vi "Muninn.vi"() -> ()   [LabVIEW 2025]
uses:
  <vilib>/OPCUA/NI OPC UA Client.lvlib
  <vilib>/Utility/config.llb/NI_LVConfig.lvlib
  <vilib>/Utility/config.llb/Read Key (String).vi
  <vilib>/OPCUA/client/Multiple Read Double.vi
panel:
  in  "Preferences Button":bool
  in  "Remove Button":bool
  in  "Add Button":bool
  in  "Sensors":i32(listbox)
  in  "Stop button":bool
  in  "Start Button":bool
  in  "LoggingIntervall":dbl=1000.0 caption="Logging intervall (ms)"
  out "running":bool
  in  "quit":bool
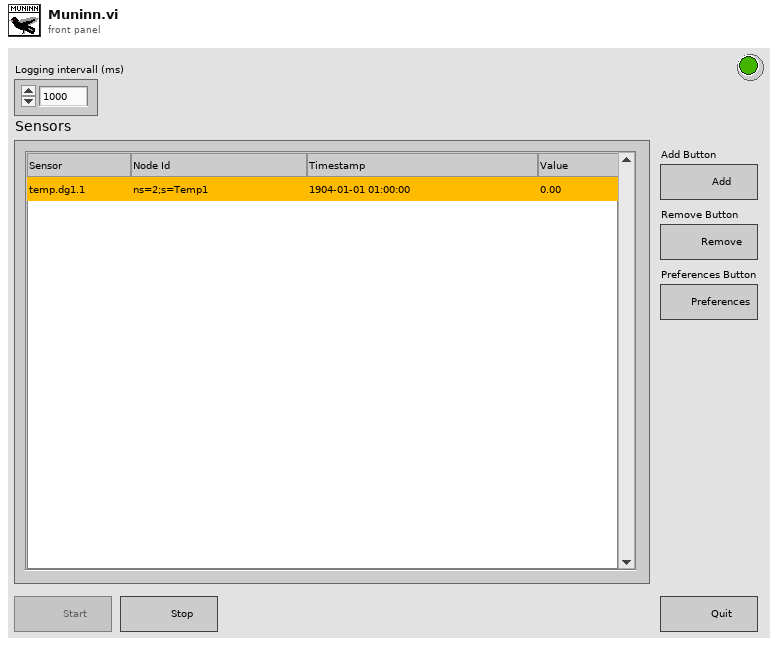
[diagram p1: front panel]
types:
  T1 = enum8{"Enabled", "Disabled", "Disabled and Grayed Out"}
  T2 = typedef "NI_LVConfig.lvlib/Config Data RefNum.ctl" = refnum<k1>
  T3 = typedef "OPC UA Client Refnum.ctl" = refnum<k21>
  T4 = typedef "NodeId.ctl" = string
  T5 = typedef "OPC UA StatusCode.ctl" = u32
  T6 = cluster{"node ID":T4, "value ":dbl, "timestamp":timestamp, "status":T5}[]
  T7 = cluster{"node ID":T4, "value ":dbl, "timestamp":timestamp, "status":T5}
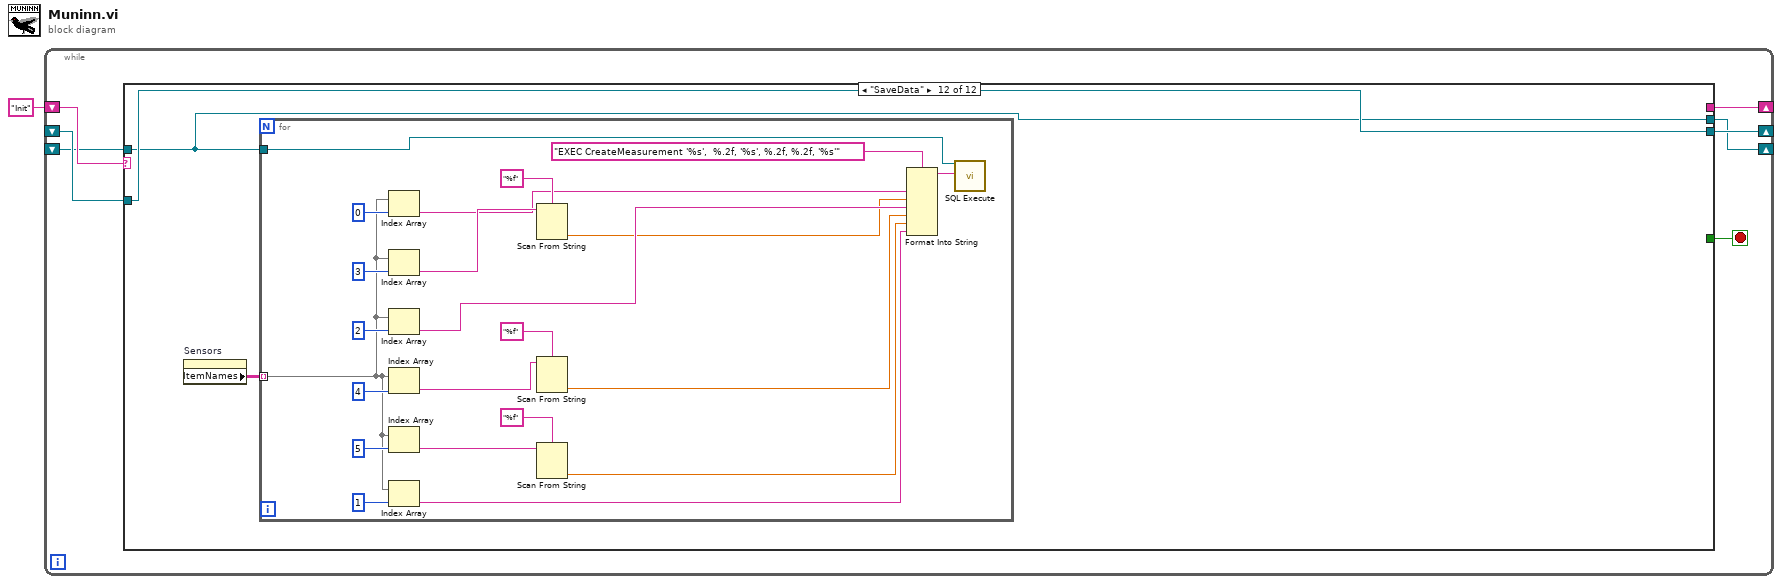
[diagram p0: block diagram]
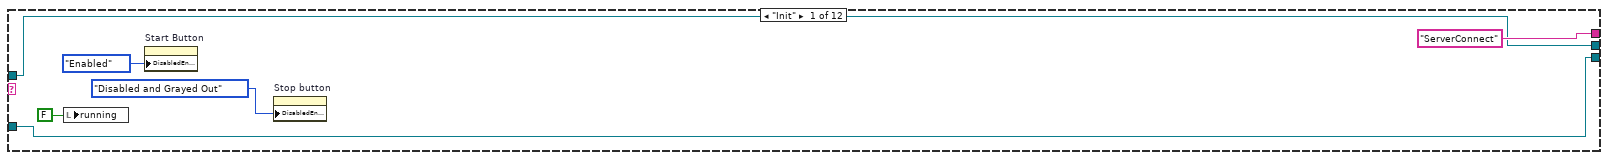
[diagram p2: hidden frame]
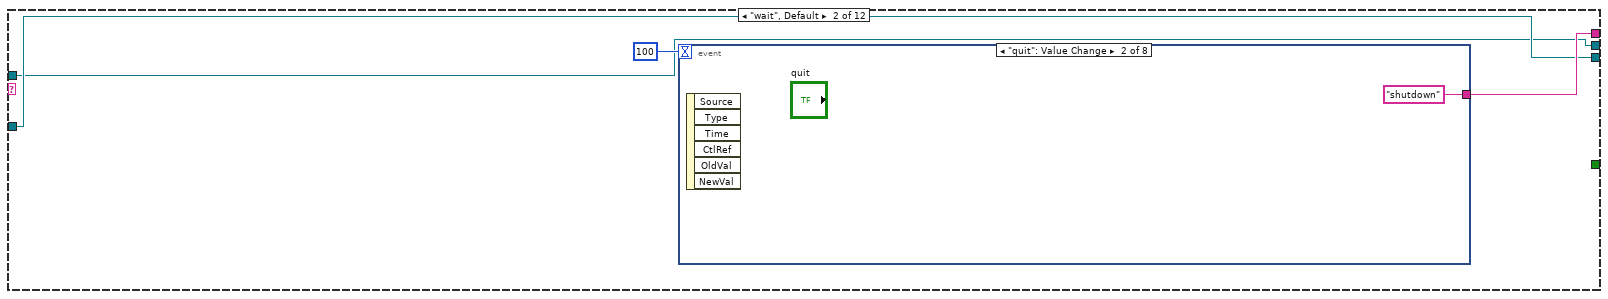
[diagram p3: hidden frame]
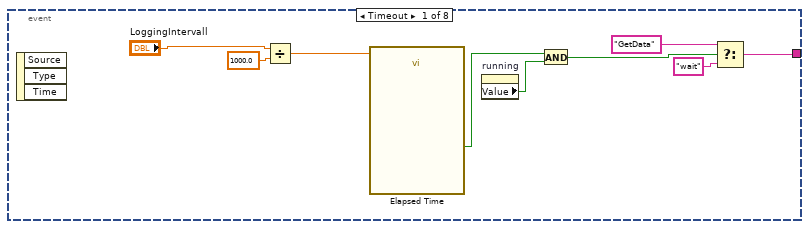
[diagram p4: hidden frame]
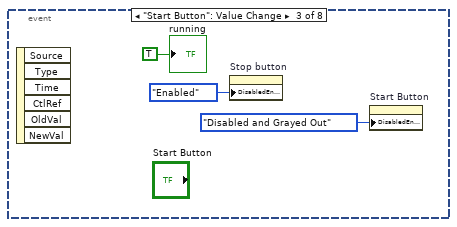
[diagram p5: hidden frame]
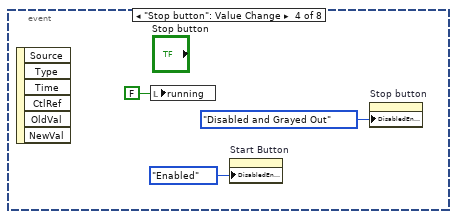
[diagram p6: hidden frame]
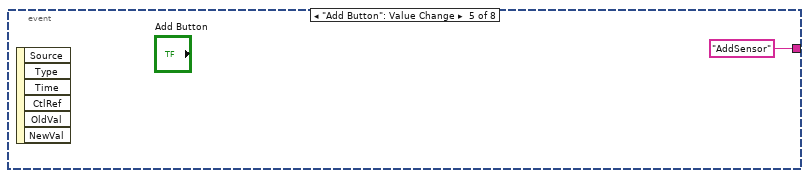
[diagram p7: hidden frame]
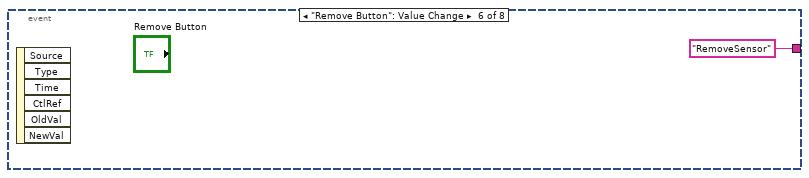
[diagram p8: hidden frame]
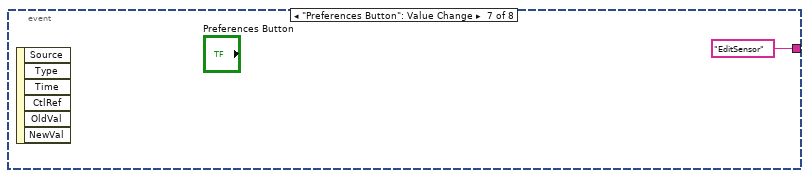
[diagram p9: hidden frame]
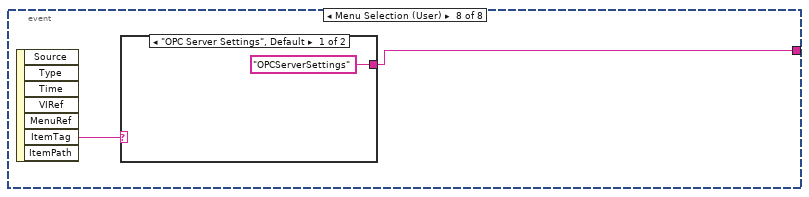
[diagram p10: hidden frame]
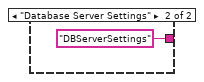
[diagram p11: hidden frame]
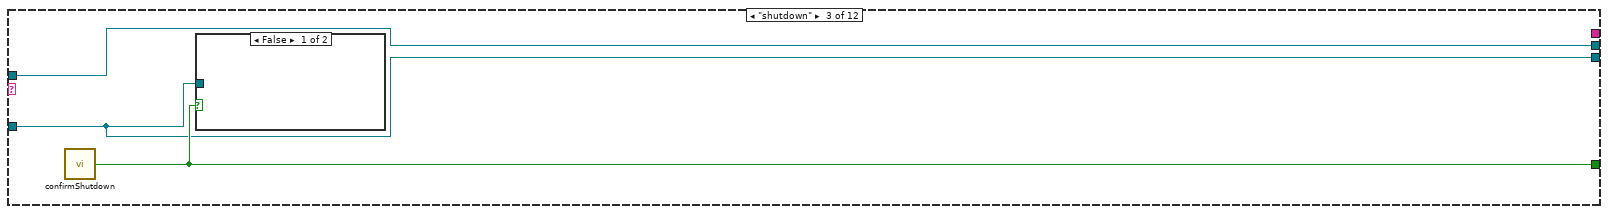
[diagram p12: hidden frame]
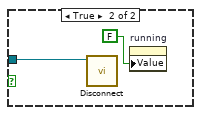
[diagram p13: hidden frame]
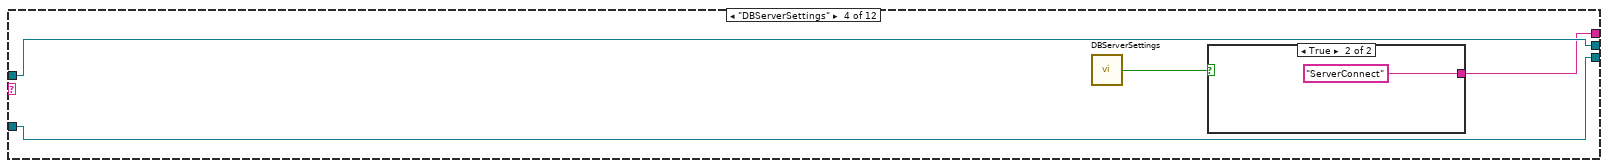
[diagram p14: hidden frame]
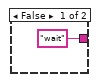
[diagram p15: hidden frame]
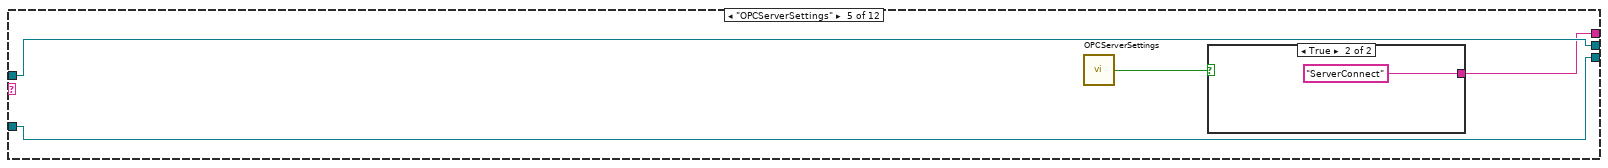
[diagram p16: hidden frame]
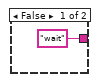
[diagram p17: hidden frame]
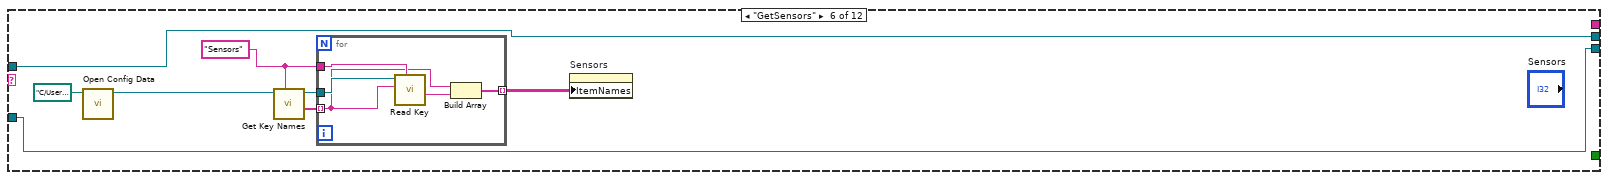
[diagram p18: hidden frame]
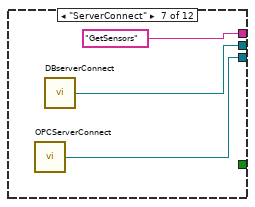
[diagram p19: hidden frame]
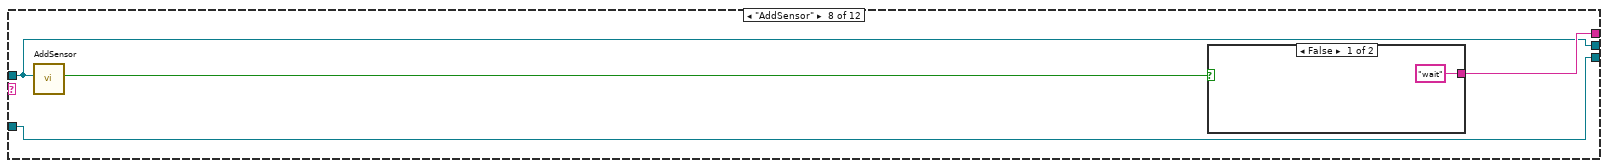
[diagram p20: hidden frame]
diagram:
  n1 = while {
    shift-right: [w7] -> _
    shift-left: "Init" -> [w8]
    shift-right: [w5] -> _
    shift-left: _ -> [w4]
    shift-right: [w3] -> _
    shift-left: _ -> [w2]
    stop <- w6 stop-if-true
    n2 = case shown="\"SaveData\"" w8 {
      tunnel: ["ServerConnect" w17 _ w48 w53 _ "GetSensors" ("t") w77 "GetSensors" ("t") w92 "SaveData" ("t") _] -> w7
      tunnel: [_ _ w44 _ _ _ _ _ _ _ _ _] -> w6
      tunnel: [w10 w16 w43 w50 w56 w66 w74 w78 w90 w95 w101 w137] -> w5
      tunnel: w4 -> [w10 w16 w43 w50 w56 w66 _ w78 w90 w95 w101 w137]
      tunnel: [w9 w15 w42 w49 w55 w59 w72 w76 w89 w94 w98 w136] -> w3
      tunnel: w2 -> [w9 w15 w42 w49 w55 w59 _ w76 w89 w94 w98 w136]
      frame "Init" {
        n3 = local write "running"(FALSE ("running")) -> ()
        n4 = property on="Start Button" class="Bool"("DisabledEnum"=T1."Enabled" ("Disabled")) -> ()  [unwired: 2 in, 2 out]
        n5 = property on="Stop button" class="Bool"("DisabledEnum"=T1."Disabled and Grayed Out" ("Disabled")) -> ()  [unwired: 2 in, 2 out]
      }
      frame "wait", Default {
        n6 = event shown="[1] \"quit\": Value Change" {
          selector: _ -> [_ _ _ _ _ _ _ _]
          dyn-events: _ -> [_ _ _ _ _ _ _ _]
          timeout: 100 -> [_ _ _ _ _ _ _ _]
          tunnel: [w25 "shutdown" ("t") _ _ "AddSensor" ("t") "RemoveSensor" ("t") "EditSensor" ("t") w39] -> w17
          event Timeout {
            n7 = event-data() -> ()  [unwired: 1 in, 3 out]
            n8 = Divide(x="LoggingIntervall", y=1000.0) -> (x/y=w20:dbl)
            n9 = call "Elapsed Time"("Time Target (s)"=w20) -> ("Time has Elapsed"=w23:bool)  [unwired: 11 in, 7 out]
            n10 = property on="running" class="Bool (strict)"() -> ("Value"=w24:bool)  [unwired: 2 in, 2 out]
            n11 = And(x=w23, y=w24) -> (x .and. y?=w27:bool)
            n12 = Select(t="GetData", s=w27, f="wait") -> (s? t:f=w25:string)
          }
          event "quit": Value Change {
            n13 = event-data() -> ()  [unwired: 1 in, 6 out]
          }
          event "Start Button": Value Change {
            n14 = event-data() -> ()  [unwired: 1 in, 6 out]
            n15 = property on="Stop button" class="Bool"("DisabledEnum"=T1."Enabled" ("Disabled")) -> ()  [unwired: 2 in, 2 out]
            n16 = property on="Start Button" class="Bool"("DisabledEnum"=T1."Disabled and Grayed Out" ("Disabled")) -> ()  [unwired: 2 in, 2 out]
            "running" <- TRUE ("running")
          }
          event "Stop button": Value Change {
            n17 = event-data() -> ()  [unwired: 1 in, 6 out]
            n18 = local write "running"(FALSE ("running")) -> ()
            n19 = property on="Start Button" class="Bool"("DisabledEnum"=T1."Enabled" ("Disabled")) -> ()  [unwired: 2 in, 2 out]
            n20 = property on="Stop button" class="Bool"("DisabledEnum"=T1."Disabled and Grayed Out" ("Disabled")) -> ()  [unwired: 2 in, 2 out]
          }
          event "Add Button": Value Change {
            n21 = event-data() -> ()  [unwired: 1 in, 6 out]
          }
          event "Remove Button": Value Change {
            n22 = event-data() -> ()  [unwired: 1 in, 6 out]
          }
          event "Preferences Button": Value Change {
            n23 = event-data() -> ()  [unwired: 1 in, 6 out]
          }
          event Menu Selection (User) {
            n24 = event-data() -> ("ItemTag"=w38:string)  [unwired: 1 in, 6 out]
            n25 = case shown="\"OPC Server Settings\", Default" w38 {
              tunnel: ["OPCServerSettings" ("t") "DBServerSettings" ("t")] -> w39
              frame "OPC Server Settings", Default {
              }
              frame "Database Server Settings" {
              }
            }
          }
        }
      }
      frame "shutdown" {
        n26 = call "confirmShutdown.vi"() -> ("OK Button 2"=w44:bool)
        n27 = case shown="False" w44 {
          tunnel: w43 -> [_ w46]
          frame False {
          }
          frame True {
            n28 = call <vilib>:"Disconnect.vi"("OPC UA client refnum in"=w46) -> ()  [unwired: 10 in, 1 out]
            n29 = property on="running" class="Bool (strict)"("Value"=FALSE ("running")) -> ()  [unwired: 2 in, 2 out]
          }
        }
      }
      frame "DBServerSettings" {
        n30 = call "DBServerSettings.vi"() -> ("OK Button 2"=w47:bool)
        n31 = case shown="True" w47 {
          tunnel: ["wait" ("t") "ServerConnect" ("t")] -> w48
          frame False {
          }
          frame True {
          }
        }
      }
      frame "OPCServerSettings" {
        n32 = call "OPCServerSettings.vi"() -> ("OK Button 2"=w54:bool)
        n33 = case shown="True" w54 {
          tunnel: ["wait" ("t") "ServerConnect" ("t")] -> w53
          frame False {
          }
          frame True {
          }
        }
      }
      frame "GetSensors" {
        w61 = "Sensors" ("section")
        n34 = call <vilib>:"Open Config Data.vi"("configuration file path"=path "C:/Users/magne/OneDrive/Dokumenter/Skole/IIA2017-1 26V Industrial Information Technology/Assignments/SCADA/02 Files/Task 3/settings.ini") -> ("refnum"=w65:T2)  [unwired: 8 in, 2 out]
        n35 = call <vilib>:"Get Key Names.vi"("section"=w61, "refnum"=w65) -> ("key names"=w63:string[], "refnum out"=w62:T2)  [unwired: 6 in, 2 out]
        n36 = for {
          tunnel: w63 -> [w68] mode=indexing
          tunnel: w62 -> [w71]
          tunnel: w61 -> [w70]
          tunnel: [w67] -> w60 mode=indexing
          n37 = call-poly <vilib>:"Read Key.vi"("section"=w70, "key"=w68, "refnum"=w71) -> ("value"=w69:string)  [unwired: 5 in, 3 out]
          n38 = Build Array(w68, w69) -> (w67:string[])
        }
        n39 = property on="Sensors" class="MCListbox (strict)"("ItemNames"=w60) -> ()  [unwired: 2 in, 2 out]
      }
      frame "ServerConnect" {
        n40 = call "OPCServerConnect.vi"() -> ("OPC UA client refnum out"=w74:T3)
        n41 = call "DBserverConnect.vi"() -> ("Connection Out"=w72:refnum<k7>)
      }
      frame "AddSensor" {
        n42 = call "AddSensor.vi"("Connection In"=w76) -> ("OK Button 2"=w75:bool)  [unwired: 10 in]
        n43 = case shown="False" w75 {
          tunnel: ["wait" ("t") "EditSensor" ("t")] -> w77
          frame False {
          }
          frame True {
          }
        }
      }
      frame "RemoveSensor" {
        n44 = property on="Sensors" class="MCListbox (strict)"() -> ("ItemNames"=w88:string[][])  [unwired: 2 in, 2 out]
        n45 = property on="Sensors" class="MCListbox (strict)"() -> ("FocusRow"=w87:i32)  [unwired: 2 in, 2 out]
        n46 = call <vilib>:"Open Config Data.vi"("configuration file path"=path "C:/Users/magne/OneDrive/Dokumenter/Skole/IIA2017-1 26V Industrial Information Technology/Assignments/SCADA/02 Files/Task 3/settings.ini") -> ("refnum"=w85:T2)  [unwired: 8 in, 2 out]
        n47 = Index Array "Index Array"(array=w88, index (row)=w87, index (col)=0) -> (element=w83:string)
        n48 = call <vilib>:"Remove Key.vi"("section"="Sensors", "key"=w83, "refnum"=w85) -> ("refnum out"=w82:T2)  [unwired: 6 in, 2 out]
        n49 = call <vilib>:"Close Config Data.vi"("refnum"=w82) -> ()  [unwired: 9 in, 2 out]
      }
      frame "EditSensor" {
        n50 = call "SensorSettings.vi"("Connection In"=w94) -> ("OK Button 2"=w93:bool)  [unwired: 2 in]
        n51 = case shown="True" w93 {
          tunnel: ["wait" ("t") "GetSensors" ("t")] -> w92
          frame False {
          }
          frame True {
          }
        }
      }
      frame "GetData" {
        n52 = property on="Sensors" class="MCListbox (strict)"() -> ("ItemNames"=w102:string[][])  [unwired: 2 in, 2 out]
        n53 = for {
          tunnel: w102 -> [w126] mode=indexing
          tunnel: w101 -> [w135]
          tunnel: [w131] -> w100 mode=indexing
          n54 = Index Array(array=w126, index=0) -> (element=w123:string)
          n55 = Index Array(array=w126, index=1) -> (element=w127:string)
          n56 = Index Array "Index Array"(array=w126, index=1) -> (element=w105:string)
          n57 = Format Into String(format string="%s.cv", w105) -> (resulting string=w116:string)  [unwired: 2 in, 1 out]
          n58 = Format Into String(format string="%s.sp", w105) -> (resulting string=w115:string)  [unwired: 2 in, 1 out]
          n59 = Build Array "Build Array"(w105, w116, w115) -> (w129:string[])
          n60 = call-poly <vilib>:"Multiple Read.vi"("node IDs"=w129, "OPC UA client refnum in"=w135) -> ("results"=w114:T6)  [unwired: 6 in, 3 out]
          n61 = Index Array "Index Array"(array=w114, index=0) -> (element=w134:T7)
          n62 = Index Array "Index Array"(array=w114, index=1) -> (element=w111:T7)
          n63 = Index Array "Index Array"(array=w114, index=2) -> (element=w110:T7)
          n64 = Unbundle By Name "Unbundle By Name"(w134) -> ("value"=w128:dbl, "timestamp"=w121:timestamp)
          n65 = Unbundle By Name "Unbundle By Name"(w111) -> ("value"=w108:dbl)
          n66 = Unbundle By Name "Unbundle By Name"(w110) -> ("value"=w109:dbl)
          n67 = Format Date/Time String(time format string (%c)="%Y-%m-%d %H:%M:%S" ("format string"), seconds (now)=w121) -> (date/time string=w119:string)  [unwired: 1 in]
          n68 = Format Into String(format string="%.2f", w128) -> (resulting string=w132:string)  [unwired: 2 in, 1 out]
          n69 = Format Into String(format string="%.2f" ("initial string"), w108) -> (resulting string=w107:string)  [unwired: 2 in, 1 out]
          n70 = Format Into String(format string="%.2f" ("initial string"), w109) -> (resulting string=w106:string)  [unwired: 2 in, 1 out]
          n71 = Build Array "Build Array"(w123, w127, w119, w132, w107, w106) -> (w131:string[])
        }
        n72 = property on="Sensors" class="MCListbox (strict)"("ItemNames"=w100) -> ()  [unwired: 2 in, 2 out]
      }
      frame "SaveData" {
        n73 = property on="Sensors" class="MCListbox (strict)"() -> ("ItemNames"=w138:string[][])  [unwired: 2 in, 2 out]
        n74 = for {
          tunnel: w138 -> [w141] mode=indexing
          tunnel: w136 -> [w156]
          n75 = Index Array "Index Array"(array=w141, index=0) -> (element=w151:string)
          n76 = Index Array "Index Array"(array=w141, index=3) -> (element=w154:string)
          n77 = Index Array "Index Array"(array=w141, index=2) -> (element=w155:string)
          n78 = Index Array "Index Array"(array=w141, index=4) -> (element=w145:string)
          n79 = Index Array "Index Array"(array=w141, index=5) -> (element=w142:string)
          n80 = Index Array "Index Array"(array=w141, index=1) -> (element=w139:string)
          n81 = Scan From String(format string="%f", input string=w154) -> (output 1=w152:dbl)  [unwired: 3 in, 3 out]
          n82 = Scan From String(format string="%f", input string=w145) -> (output 1=w143:dbl)  [unwired: 3 in, 3 out]
          n83 = Scan From String(format string="%f", input string=w142) -> (output 1=w144:dbl)  [unwired: 3 in, 3 out]
          n84 = Format Into String(format string="EXEC CreateMeasurement '%s',  %.2f, '%s', %.2f, %.2f, '%s'", w151, w152, w155, w143, w144, w139) -> (resulting string=w150:string)  [unwired: 2 in, 1 out]
          n85 = call <vilib>:"SQL Execute.vi"("Connection In"=w156, "SQL Query"=w150) -> ()  [unwired: 16 in, 2 out]
        }
      }
    }
  }
